vi "rsmxo_LV2015_Read_Device_IDN_Example.vi"() -> ()   [LabVIEW 2015]
uses:
  <instrlib>/Rohde&Schwarz MXO Oscilloscopes/Rohde&Schwarz MXO Oscilloscopes.lvlib
panel:
  out "*IDN? response":string
  in  "VISA resource name":refnum<visa-resource-name>="TCPIP::10.112.0.157::hislip0"
  in  "Reset":bool
  in  "ID Query":bool=TRUE
  # "Rohde & Schwarz MXO Oscilloscopes Series\n*IDN? Example"
  # "Before running, change the VISA resource name to fit your device:\n- For LAN interface use TCPIP::<IP_Address>::INSTR e.g. TCPIP::10.64.0.178::INSTR\n- For USB interface use USB0::0x0AAD::<PID>::<SN>::INSTR e.g. USB0::0x0AAD::0x01D6::101457::INSTR\n- For GPIB interface use the GPIB::<Address>::INSTR e.g. GPIB::28::INSTR"
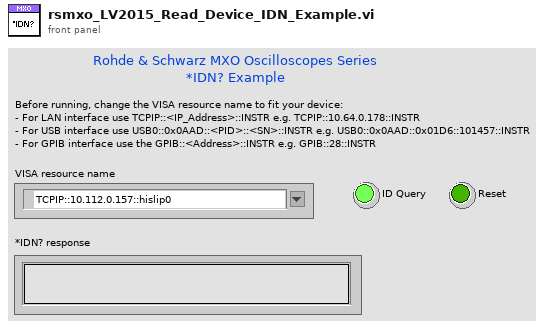
[diagram p1: front panel]
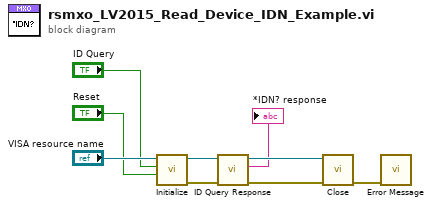
[diagram p0: block diagram]
diagram:
  n1 = call <instrlib>:"Initialize.vi"("Reset (T: Reset)"="Reset", "ID Query (T: Check)"="ID Query", "VISA resource name"="VISA resource name") -> ("error out"=w5:errorcluster, "VISA resource name out"=w4:refnum<visa-resource-name>)  [unwired: 7 in]
  n2 = call <instrlib>:"ID Query Response.vi"("error in (no error)"=w5, "VISA resource name"=w4) -> ("error out"=w3:errorcluster, "ID Query Response"=→"*IDN? response":string, "VISA resource name out"=w2:refnum<visa-resource-name>)  [unwired: 7 in]
  n3 = call <instrlib>:"Close.vi"("error in (no error)"=w3, "VISA resource name"=w2) -> ("error out"=w6:errorcluster)  [unwired: 9 in]
  n4 = call <instrlib>:"Error Message.vi"("error in (no error)"=w6) -> ()  [unwired: 10 in, 5 out]
